vi "Configure Frequency.vi"(7 "Mode":enum16{"Center Span", "Start Stop"}(ring), 8 "error in (no error)":errorcluster, 9 "Span/Stop Frequency":dbl, 10 "Center/Start Frequency":dbl, 11 "VNA-CMT S2 S4 in":refnum<class "VNA-CMT S2 S4.lvclass">) -> (0 "error out":errorcluster, 3 "VNA-CMT S2 S4 out":refnum<class "VNA-CMT S2 S4.lvclass">)   [LabVIEW 2020, in "VNA-CMT S2 S4.lvclass"]
doc: "Configures the frequency range for the sweep.\nThe default mode is Center Span."
uses:
  VNA-CMT S2 S4.lvclass
  C:/Sandbox/Git_Sandbox/WiSpry Test Framework source code (LV20)/WiSpry Test Framework/Instruments/Instrument.lvclass
  Instrument.lvclass/Instrument.ctl
  Instrument.lvclass
  <instrlib>/CMT S2 and S4 VNA/CMT S2 and S4 VNA.lvlib
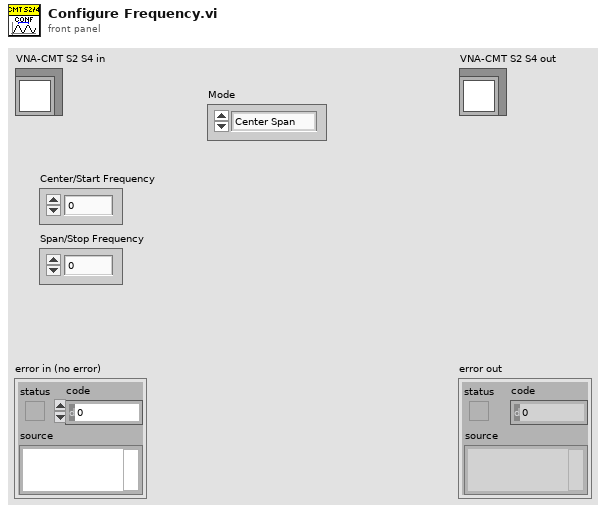
[diagram p1: front panel]
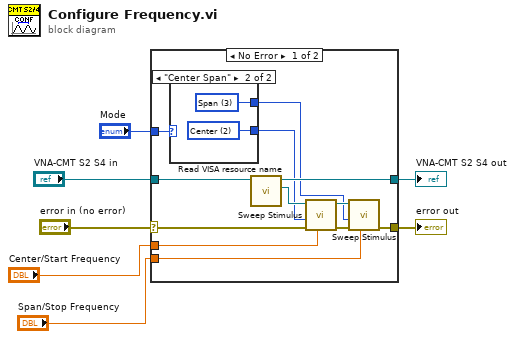
[diagram p0: block diagram]
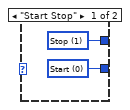
[diagram p2: hidden frame]
diagram:
  n1 = case shown="No Error" "error in (no error)" {
    selector: "error in (no error)" -> [w8 w24]
    tunnel: "VNA-CMT S2 S4 in" -> [w19 w25]
    tunnel: [w18 w25] -> w5
    tunnel: [w9 w24] -> w6
    tunnel: "Center/Start Frequency" -> [w16 _]
    tunnel: "Mode" -> [w11 _]
    tunnel: "Span/Stop Frequency" -> [w10 _]
    frame No Error {
      n2 = case shown="\"Center Span\"" w11 {
        tunnel: [w21 w23] -> w15
        tunnel: [w20 w22] -> w12
        frame "Start Stop" {
          w20 = u16 1 items=["Start", "Stop", "Center", "Span"] ("Stimulus (0: Start)")
          w21 = u16 0 items=["Start", "Stop", "Center", "Span"] ("Stimulus (0: Start)")
        }
        frame "Center Span" {
          w22 = u16 3 items=["Start", "Stop", "Center", "Span"] ("Stimulus (0: Start)")
          w23 = u16 2 items=["Start", "Stop", "Center", "Span"] ("Stimulus (0: Start)")
        }
      }
      n3 = call "Read VISA resource name.vi"("Instrument in"=w19) -> ("VISA resource name"=w17:refnum<visa-resource-name>, "Instrument out"=w18:refnum<class "VNA-CMT S2 S4.lvclass">)  [unwired: 9 in]
      n4 = call <instrlib>:"Sweep Stimulus.vi"("Parameter (0.0)"=w16, "error in (no error)"=w8, "Stimulus (0: Start)"=w15, "VISA resource name"=w17) -> ("error out"=w14:errorcluster, "VISA resource name out"=w13:refnum<visa-resource-name>)  [unwired: 6 in]
      n5 = call <instrlib>:"Sweep Stimulus.vi"("Parameter (0.0)"=w10, "error in (no error)"=w14, "Stimulus (0: Start)"=w12, "VISA resource name"=w13) -> ("error out"=w9:errorcluster)  [unwired: 6 in, 1 out]
    }
    frame Error {
    }
  }
  "error out" <- w6
  "VNA-CMT S2 S4 out" <- w5
